vi "T7 Byte to Volts KAG.vi"(8 "error in":errorcluster, 11 "Byte Data":u16[][](array[numeric])) -> (0 "error out":errorcluster, 3 "Float Data":dbl[][](array[numeric]))   [LabVIEW 2022 SP3]
doc: "Apply T7 calibration contents (read from flash memory chip) to convert U16 data to raw voltage data.\n\nThere is a plot on the right hidden by the front panel edge."
uses:
  T7 Stream Globals KAG.vi
panel:
  out "Waveform Graph":dbl[][](graph)
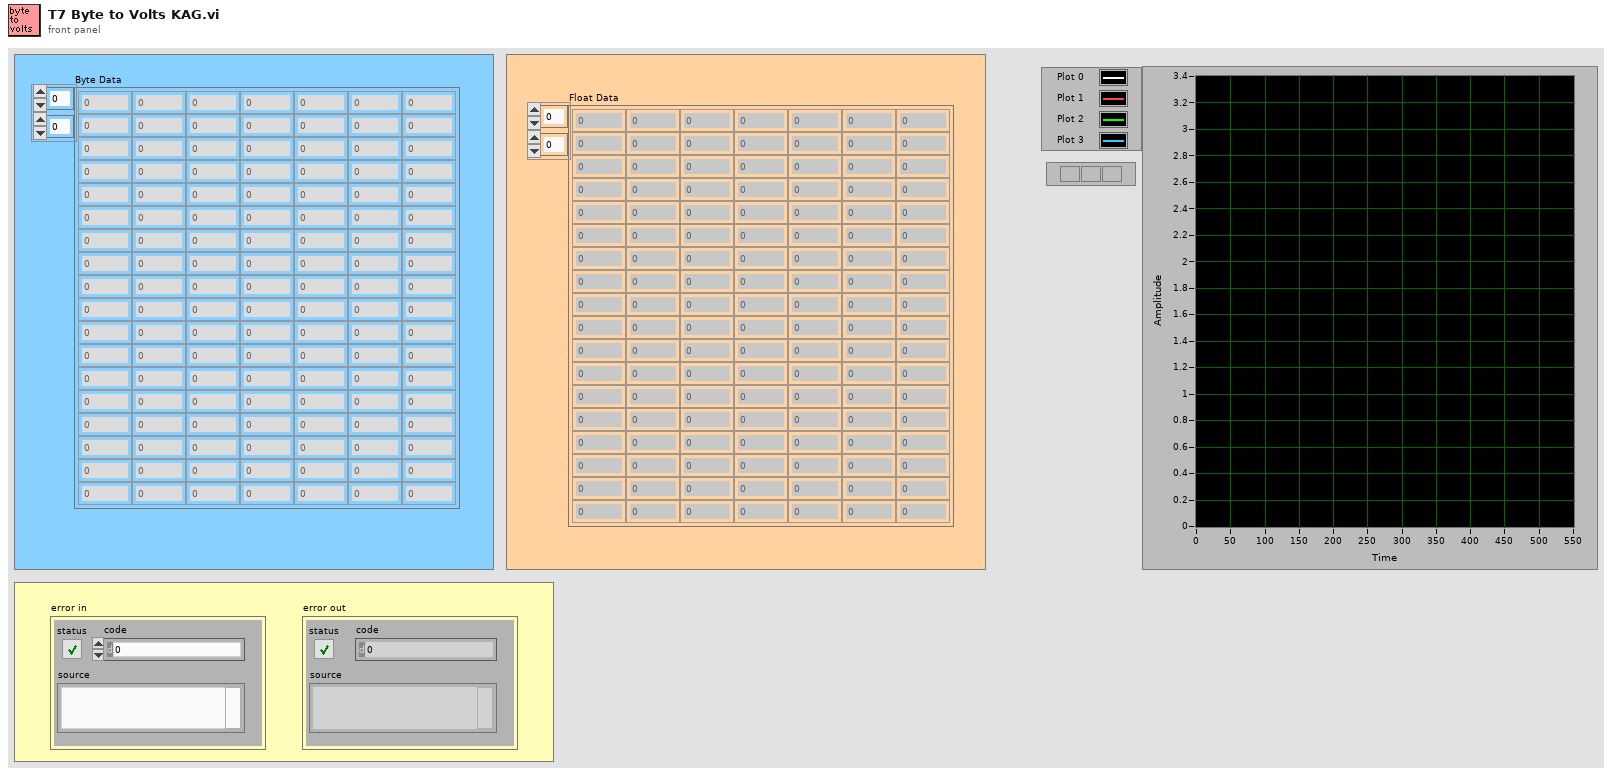
[diagram p1: front panel]
types:
  T1 = cluster{"Channel":u32, "BipGain":u32, "Input Config":string}[]
  T2 = cluster{"PSlope":dbl, "NSlope":dbl, "AvgSlope":dbl, "Center":dbl, "Offset":dbl}[]
  T3 = cluster{"PSlope":dbl, "NSlope":dbl, "AvgSlope":dbl, "Center":dbl, "Offset":dbl}
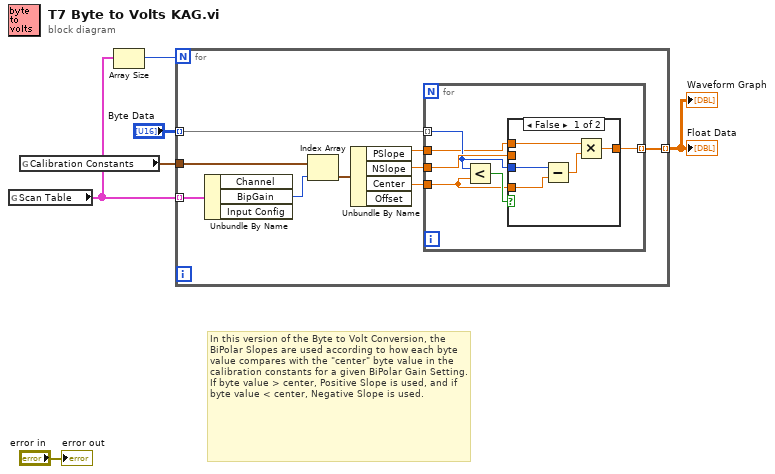
[diagram p0: block diagram]
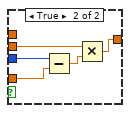
[diagram p2: hidden frame]
diagram:
  # "In this version of the Byte to Volt Conversion, the BiPolar Slopes are used according to how each byte value compares with the \"center\" byte value in the calibration constants for a given BiPolar Gain Setting. If byte value > center, Positive Slope is used, and if byte value < center, Negative Slope is used."
  n1 = global read "T7 Stream Globals KAG.vi" "Scan Table"() -> (w6:T1)
  n2 = global read "T7 Stream Globals KAG.vi" "Calibration Constants"() -> (w4:T2)
  n3 = Array Size(array=w6) -> (size(s)=w5:i32)
  n4 = for {
    N: w5 -> [_]
    tunnel: w6 -> [w15] mode=indexing
    tunnel: w4 -> [w14]
    tunnel: "Byte Data" -> [w7] mode=indexing
    tunnel: [w8] -> w1 mode=indexing
    n5 = Unbundle By Name(w15) -> ("BipGain"=w12:u32)  [unwired: 2 out]
    n6 = Index Array(array=w14, index=w12) -> (element=w13:T3)
    n7 = Unbundle By Name(w13) -> ("PSlope"=w9:dbl, "NSlope"=w10:dbl, "Center"=w11:dbl)  [unwired: 1 out]
    n8 = for {
      tunnel: w7 -> [w19] mode=indexing
      tunnel: w11 -> [w18]
      tunnel: w10 -> [w20]
      tunnel: w9 -> [w17]
      tunnel: [w16] -> w8 mode=indexing
      n9 = Less?(x=w19, y=w18) -> (x < y?=w21:bool)
      n10 = case shown="False" w21 {
        tunnel: w20 -> [_ w28]
        tunnel: w19 -> [w25 w31]
        tunnel: w18 -> [w24 w30]
        tunnel: [w23 w27] -> w16
        tunnel: w17 -> [w26 _]
        frame False {
          n11 = Subtract(x=w25, y=w24) -> (x-y=w22:dbl)
          n12 = Multiply(x=w26, y=w22) -> (x*y=w23:dbl)
        }
        frame True {
          n13 = Subtract(x=w31, y=w30) -> (x-y=w29:dbl)
          n14 = Multiply(x=w28, y=w29) -> (x*y=w27:dbl)
        }
      }
    }
  }
  "Float Data" <- w1
  "Waveform Graph" <- w1
  "error out" <- "error in"
